vi "GA Get Look Ahead Space.vi"(8 "error in (no error)":errorcluster caption="错误输入（无错误）", 9 "nFifoIndex":i16, 10 "pSpace":i32, 11 "nCrdNum":i16) -> (0 "error out":errorcluster caption="错误输出", 2 "pSpace out":i32, 3 "function return":i32)   [LabVIEW 2015, in "GAS.lvlib"]
doc: "extern \"C\" __declspec(dllimport) int GA_GetLookAheadSpace(short nCrdNum,long *pSpace,short nFifoIndex=0);"
uses:
  <userlib>/BP_GAS/GAS.lvlib
  <userlib>/BP_GAS/GAS.dll
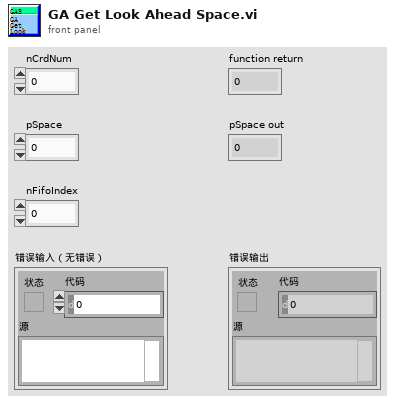
[diagram p1: front panel]
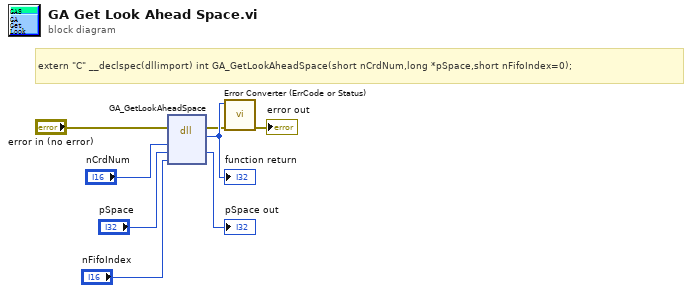
[diagram p0: block diagram]
diagram:
  # "extern \"C\" __declspec(dllimport) int GA_GetLookAheadSpace(short nCrdNum,long *pSpace,short nFifoIndex=0);"
  n1 = dll-call lib="E:/Program Files (x86)/National Instruments/LabVIEW 2015/user.lib/BP_GAS/GAS.*" fn="GA_GetLookAheadSpace"(error in="error in (no error)", "nCrdNum"="nCrdNum", "pSpace"="pSpace", "nFifoIndex"="nFifoIndex") -> (error out=w2:errorcluster, w8:i32, "pSpace"=→"pSpace out":i32)  [unwired: 4 in, 1 out]
  "function return" <- w8
  n2 = call "Error Converter (ErrCode or Status).vi"("error in (no error)"=w2, "error code"=w8) -> ("error out"=→"error out":errorcluster)  [unwired: 9 in]
